vi "Spartan Server Startup.vi"(8 "error in (no error)":errorcluster, 11 "Version":T1={"Version"="", "Build Number"=0, "Build Date/Time"=-9593222399.39995} {"Build Date/Time" format="%<%X\n%x>T"}) -> (0 "error out":errorcluster, 2 "DIAdem?":bool)   [LabVIEW 2011]
uses:
  SI.LIB/OGAB Version.ctl
panel:
  out "bigver":string
  out "version status":string
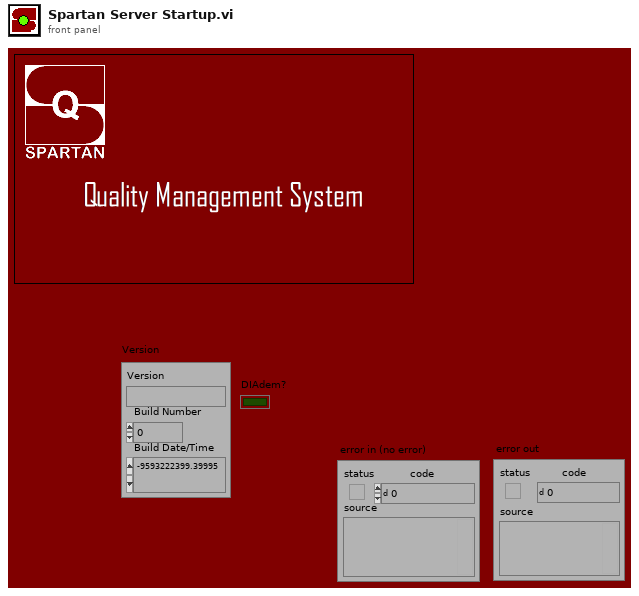
[diagram p1: front panel]
types:
  T1 = typedef "OGAB Version.ctl" = cluster{"Version":string, "Build Number":u32, "Build Date/Time":dbl}
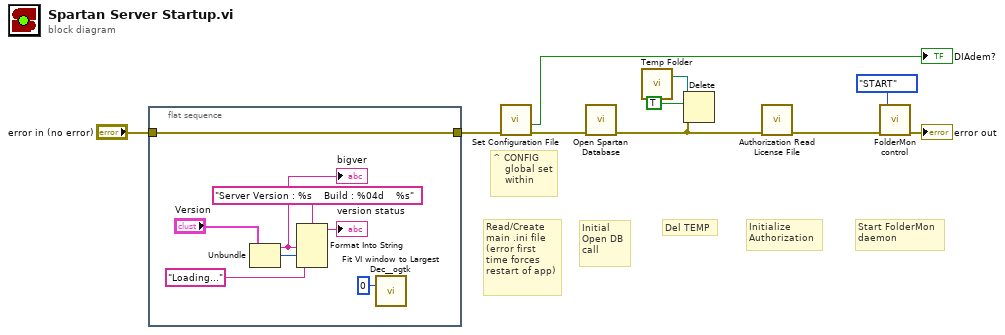
[diagram p0: block diagram]
diagram:
  # "Initialize\nAuthorization"
  # "Initial \nOpen DB\ncall"
  # "Del TEMP"
  # "^ CONFIG\n    global set\n    within"
  # "Read/Create\nmain .ini file\n(error first\ntime forces\nrestart of app)"
  # "Start FolderMon\ndaemon"
  n1 = flat-sequence {
    tunnel: "error in (no error)" -> [w11]
    tunnel: [w11] -> w5
    frame #0 {
      n2 = Unbundle("Version") -> ("Version"=w14:string, "Build Number"=w16:u32)  [unwired: 1 out]
      "bigver" <- w14
      n3 = Format Into String(format string="Server Version : %s    Build : %04d    %s", w14, w16, "Loading..." ("format string")) -> (resulting string=→"version status":string)  [unwired: 2 in, 1 out]
      n4 = call "Fit VI window to Largest Dec__ogtk.vi"("border spacing (2 px)"=0) -> ()  [unwired: 2 in, 5 out]
    }
  }
  n5 = call "Set Configuration File.vi"("error in (no error)"=w5) -> ("error out"=w6:errorcluster, "DIAdem?"=→"DIAdem?":bool)  [unwired: 9 in]
  n6 = call "Open Spartan Database.vi"("error in (no error)"=w6) -> ("error out"=w2:errorcluster)  [unwired: 9 in, 1 out]
  n7 = call "Temp Folder.vi"() -> ("Temp Folder"=w7:path)  [unwired: 3 in]
  n8 = Delete(path (use dialog)=w7, entire hierarchy (F)=TRUE, error in=w2) -> ()  [unwired: 5 out]
  n9 = call "Authorization Read License File.vi"("error in (no error)"=w2) -> ("error out"=w1:errorcluster)  [unwired: 9 in, 1 out]
  n10 = call "FolderMon control.vi"("error in (no error)"=w1, "Action (START)"=enum16{"START", "STOP"}."START") -> ("error out"=→"error out":errorcluster)  [unwired: 1 in, 4 out]
